vi "Parameters File Handler.vi"(8 "error in":errorcluster, 10 "selected parameters file":path caption="path to parameters xml", 11 "configuration files page data":T1 {"custom device ref" format="%.0x"}) -> (0 "error out":errorcluster, 3 "configuration files page data out":T1 {"custom device ref" format="%.0x"})   [LabVIEW 2020, in "AIM ARINC 429 System Explorer.lvlib" / "Implementation.lvlib"]
uses:
  Implementation.lvlib
  Types/Configuration Files Page Data.ctl
  Types/Path Control.ctl
  Types/Browse Button.ctl
  <vilib>/NI VeriStand/Custom Device API/Custom Device Item Ref.ctl
  Import/ARINC 429 Import.lvlib
  Scripting/AIM/AIM ARINC 429 Scripting.lvlib
  <vilib>/NI VeriStand/Custom Device API/Custom Device API.lvlib
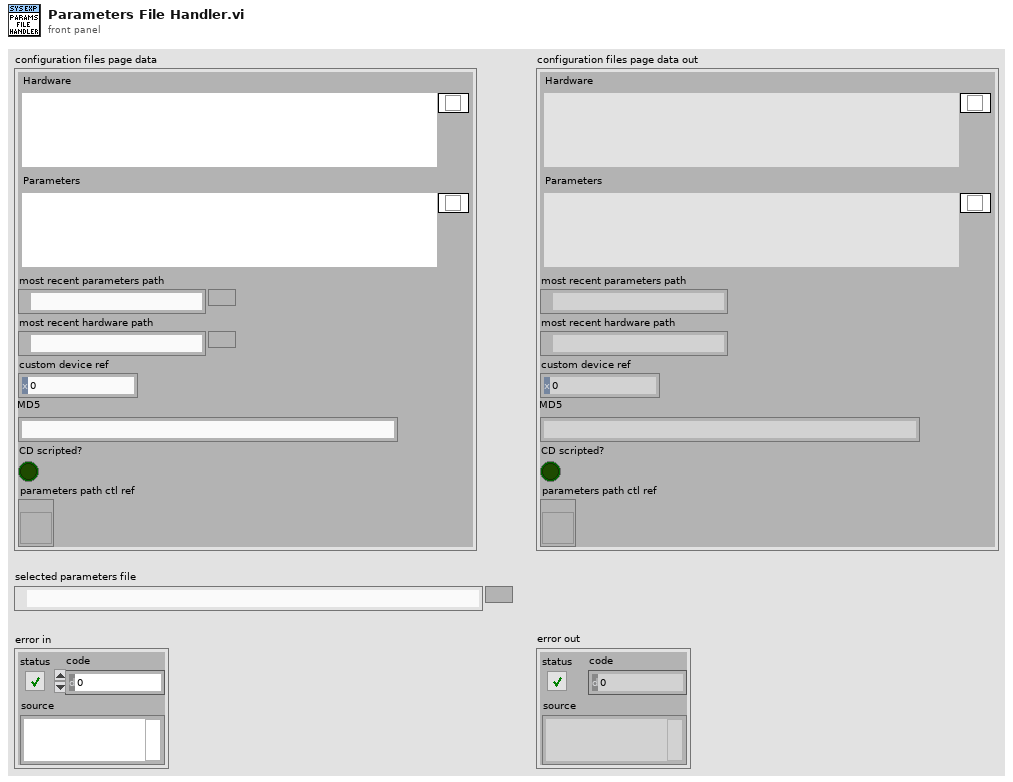
[diagram p1: front panel]
types:
  T1 = typedef "AIM ARINC 429 System Explorer.lvlib/Implementation.lvlib/Configuration Files Page Data.ctl" = cluster{"Hardware":T2, "Parameters":T2, "most recent parameters path":path, "most recent hardware path":path, "custom device ref":T4, "MD5":string, "CD scripted?":bool, "parameters path ctl ref":refnum<vi>}
  T2 = typedef "AIM ARINC 429 System Explorer.lvlib/Implementation.lvlib/Path Control.ctl" = cluster{"file path":path, "Browse":T3}
  T3 = typedef "AIM ARINC 429 System Explorer.lvlib/Implementation.lvlib/Browse Button.ctl" = bool
  T4 = typedef "Custom Device API.lvlib/Custom Device Item Ref.ctl" = u64
  T5 = typedef "VS Channels Definition for All Labels on Hardware Channel.ctl" = cluster{"hardware channel":i32, "direction":T6, "labels":T7[]}
  T6 = typedef "Direction.ctl" = enum16{"Rx", "Tx"}
  T7 = typedef "VS Channels Definition for Label.ctl" = cluster{"label (Dec)":u32, "parameters":T8[], "SDI value":u8, "SDI enabled":bool, "transfer type":T11, "create timestamp":bool}
  T8 = typedef "VS Channel Definition for Parameter.ctl" = cluster{"name":string, "default value":dbl, "unit":string, "Parameter":T9}
  T9 = typedef "Parameter Definition.ctl" = cluster{"start index":i32, "size":i32, "encoding":T10, "signed":bool, "scale multiplier":dbl, "scale offset":dbl}
  T10 = typedef "Encoding and Decoding.lvlib/Encoding.ctl" = enum16{"BNR", "BCD", "Discrete"}
  T11 = typedef "Transfer Type.ctl" = enum16{"Scheduled", "Acyclic", "Block", "Strobe"}
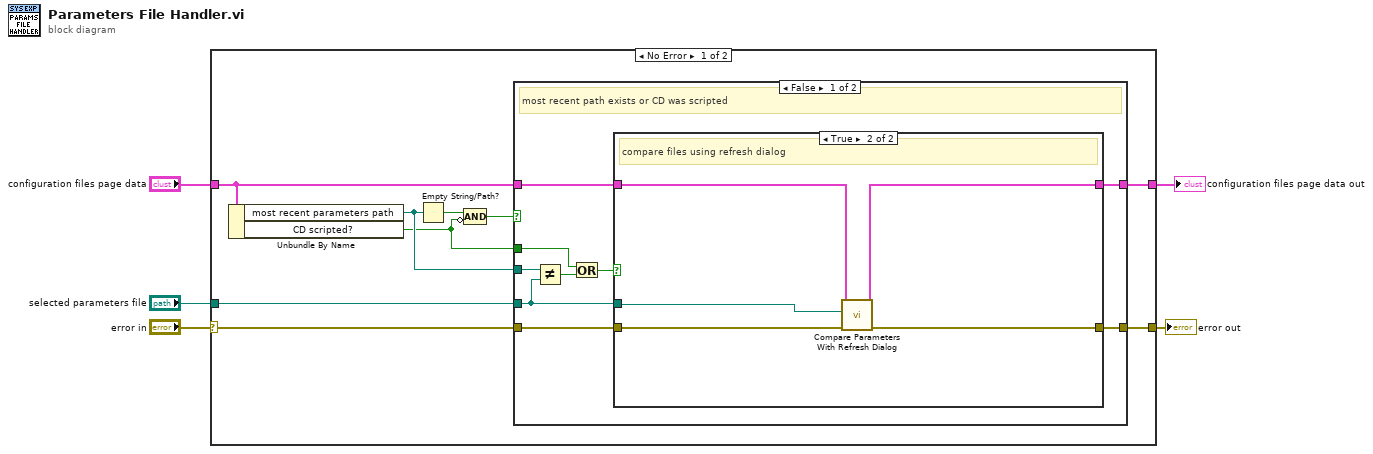
[diagram p0: block diagram]
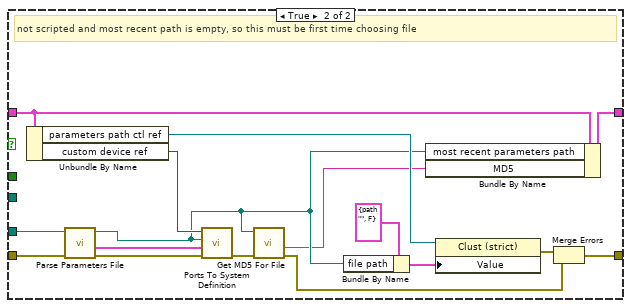
[diagram p3: hidden frame]
diagram:
  n1 = case shown="No Error" "error in" {
    selector: "error in" -> [w14 w48]
    tunnel: [w13 w48] -> w4
    tunnel: "configuration files page data" -> [w11 w47]
    tunnel: [w10 w47] -> w2
    tunnel: "selected parameters file" -> [w12 _]
    frame No Error {
      n2 = Unbundle By Name(w11) -> ("most recent parameters path"=w9:path, "CD scripted?"=w6:bool)
      n3 = Empty String/Path?(string/path=w9) -> (empty?=w8:bool)
      n4 = Compound Arithmetic op=AND(w8, invert w6) -> (w7:bool)
      n5 = case shown="False" w7 {
        tunnel: w14 -> [w23 w46]
        tunnel: w12 -> [w22 w45]
        tunnel: [w21 w38] -> w13
        tunnel: w9 -> [w20 _]
        tunnel: w11 -> [w19 w37]
        tunnel: [w18 w36] -> w10
        tunnel: w6 -> [w15 _]
        frame False {
          # "most recent path exists or CD was scripted"
          n6 = Not Equal?(x=w20, y=w22) -> (x != y?=w17:bool)
          n7 = Or(x=w15, y=w17) -> (x .or. y?=w16:bool)
          n8 = case shown="True" w16 {
            tunnel: w23 -> [w25 w30]
            tunnel: w22 -> [_ w26]
            tunnel: [w25 w27] -> w21
            tunnel: w19 -> [w24 w29]
            tunnel: [w24 w28] -> w18
            frame False {
              # "same path and CD not scripted, so do nothing"
            }
            frame True {
              # "compare files using refresh dialog"
              n9 = call "Compare Parameters With Refresh Dialog.vi"("error in"=w30, "selected parameters file"=w26, "configuration files page data"=w29) -> ("error out"=w27:errorcluster, "configuration files page data out"=w28:T1)  [unwired: 7 in]
            }
          }
        }
        frame True {
          # "not scripted and most recent path is empty, so this must be first time choosing file"
          n10 = Unbundle By Name(w37) -> ("parameters path ctl ref"=w35:refnum<vi>, "custom device ref"=w42:T4)
          n11 = call "Parse Parameters File.vi"("error in"=w46, "path to XML document"=w45) -> ("error out"=w44:errorcluster, "ports"=w43:T5[], "path to XML document out"=w32:path)  [unwired: 7 in]
          n12 = call "Ports To System Definition.vi"("error in"=w44, "ports"=w43, "parameter configuration file path"=w32, "custom device ref"=w42) -> ("error out"=w34:errorcluster)  [unwired: 6 in, 1 out]
          n13 = call "Get MD5 For File.vi"("error in"=w34, "path"=w32) -> ("error out"=w33:errorcluster, "MD5"=w31:string)  [unwired: 8 in]
          n14 = Bundle By Name(cluster=T2 {"file path"=path "", "Browse"=FALSE} ("Value"), "file path"=w32) -> (w41:T2)
          n15 = Bundle By Name(cluster=w37, "most recent parameters path"=w32, "MD5"=w31) -> (w36:T1)
          n16 = property class="Clust (strict)"(reference=w35, "Value"=w41) -> (error out=w39:errorcluster)  [unwired: 1 in, 1 out]
          n17 = Merge Errors(w39, w33) -> (w38:errorcluster)
        }
      }
    }
    frame Error {
    }
  }
  "error out" <- w4
  "configuration files page data out" <- w2
